vi "Helper SubVI - Get Single-level Approximation Coefficients.vi"(9 "index of Lengths":i32, 10 "Lengths":i32[](array[numeric]), 11 "DWT":dbl[](array[numeric])) -> (1 "left length":i32, 2 "Lengths out":i32[](array[numeric]), 3 "DWT 2":dbl[](array[numeric]))   [LabVIEW 2023]
doc: "Gets the single-level approximation coefficients."
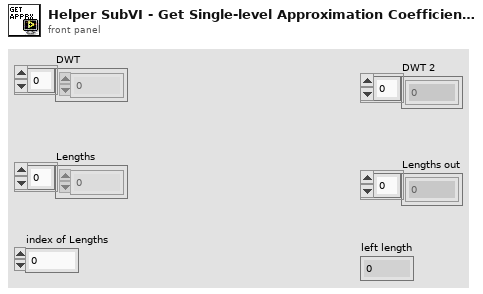
[diagram p1: front panel]
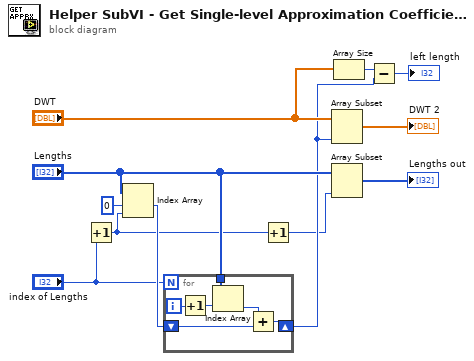
[diagram p0: block diagram]
diagram:
  n1 = Increment(x="index of Lengths") -> (x+1=w8:i32)
  n2 = Index Array(array="Lengths", index #1=0 ("index"), index #2=w8) -> (element #1=w12:i32)  [unwired: 1 out]
  n3 = for {
    N: "index of Lengths" -> [_]
    shift-right: [w13] -> w3
    shift-left: w12 -> [w14]
    tunnel: "Lengths" -> [w18]
    i -> [w17]
    n4 = Increment(x=w17) -> (x+1=w16:i32)
    n5 = Index Array(array=w18, index=w16) -> (element=w15:i32)
    n6 = Add(x=w15, y=w14) -> (x+y=w13:i32)
  }
  n7 = Increment(x=w8) -> (x+1=w1:i32)
  n8 = Array Subset(array="DWT", length=w3) -> (→"DWT 2":dbl[])  [unwired: 1 in]
  n9 = Array Subset(array="Lengths", length=w1) -> (→"Lengths out":i32[])  [unwired: 1 in]
  n10 = Array Size(array="DWT") -> (size(s)=w4:i32)
  n11 = Subtract(x=w4, y=w3) -> (x-y=→"left length":i32)
